vi "PhotonPipelineResult_HasTargets.vi"(11 "PhotonPipelineResult":T1 {"Targets"."Pose"."ROTATION"."SIN" format="%13.4f"; "Targets"."Pose"."ROTATION"."COS" format="%13.4f"; "Targets"."Pose"."ROTATION"."VALUE" format="%13.4f"; "Targets"."Pose"."TRANSLATION"."Y" format="%14.3f"; "Targets"."Pose"."TRANSLATION"."X" format="%14.3f"}) -> (3 "HasTargets":bool)   [LabVIEW 2019, in "PhotonVisionLib.lvlib"]
doc: "Returns whether the pipeline has targets.\n\nInputs:\n - PipelineResult -- Parsed PipelineResult cluster.\n\nOutputs:\n - HasTargets -- Whether the pipeline has targets."
uses:
  TypeDef/PhotonPipelineResultType.ctl
  PhotonVisionLib.lvlib
  TypeDef/TargetCornerType.ctl
  TypeDef/PhotonTrackedTargetType.ctl
  <vilib>/Rock Robotics/WPI/ThirdParty/JAS_Junk/TrajLib/TRANSLATION2D.ctl
  <vilib>/Rock Robotics/WPI/ThirdParty/JAS_Junk/TrajLib/Trajectory_Library.lvlib
  <vilib>/Rock Robotics/WPI/ThirdParty/JAS_Junk/TrajLib/ROTATION2D.ctl
  <vilib>/Rock Robotics/WPI/ThirdParty/JAS_Junk/TrajLib/POSE2D.ctl
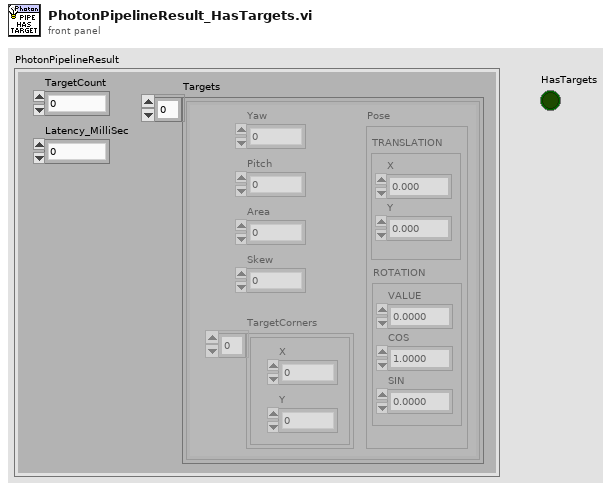
[diagram p1: front panel]
types:
  T1 = typedef "PhotonVisionLib.lvlib/PhotonPipelineResultType.ctl" = cluster{"TargetCount":i32, "Latency_MilliSec":dbl, "Targets":T2[]}
  T2 = typedef "PhotonVisionLib.lvlib/PhotonTrackedTargetType.ctl" = cluster{"Yaw":dbl, "Pitch":dbl, "Area":dbl, "Skew":dbl, "TargetCorners":T3[], "Pose":T4}
  T3 = typedef "PhotonVisionLib.lvlib/TargetCornerType.ctl" = cluster{"X":dbl, "Y":dbl}
  T4 = typedef "Trajectory_Library.lvlib/POSE2D.ctl" = cluster{"TRANSLATION":T5, "ROTATION":T6}
  T5 = typedef "Trajectory_Library.lvlib/TRANSLATION2D.ctl" = cluster{"X":dbl, "Y":dbl}
  T6 = typedef "Trajectory_Library.lvlib/ROTATION2D.ctl" = cluster{"VALUE":dbl, "COS":dbl, "SIN":dbl}
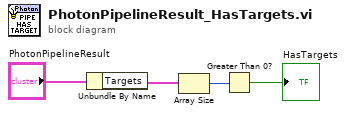
[diagram p0: block diagram]
diagram:
  n1 = Unbundle By Name("PhotonPipelineResult") -> ("Targets"=w2:T2[])
  n2 = Array Size(array=w2) -> (size(s)=w3:i32)
  n3 = Greater Than 0?(x=w3) -> (x > 0?=→"HasTargets":bool)
